vi "GrabFullListing.vi"(10 "Device In":T1, 11 "MulticolumnListbox in":refnum<vi>) -> (2 "tags":string[](array[string]))   [LabVIEW 2016, in "Systemlink Tag.xctl"]
uses:
  <userlib>/MicroPython/VIs/SystemLink/Systemlink Tag.xctl
  <userlib>/MicroPython/VIs/SystemLink/SkylineCluster.ctl
panel:
  out "Table Control":string[][](table)
  out "error out":errorcluster
  in  "error in":errorcluster
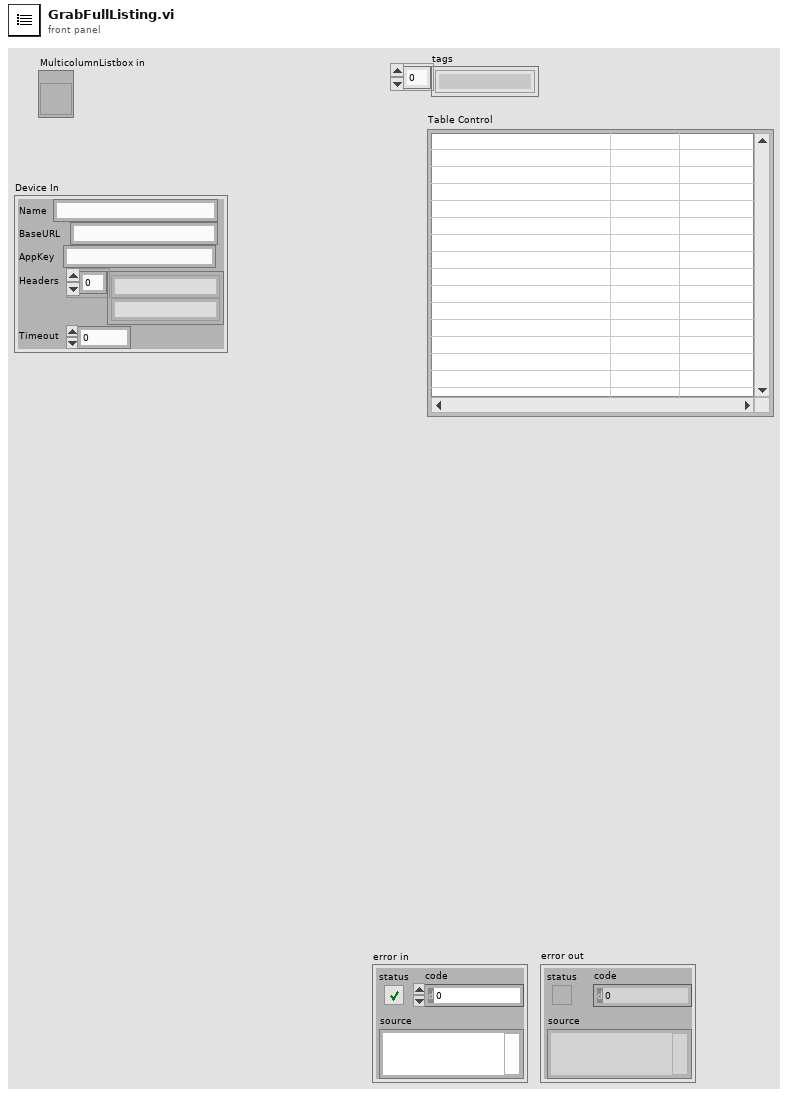
[diagram p1: front panel]
types:
  T1 = typedef "SkylineCluster.ctl" = cluster{"Name":string, "BaseURL":string, "AppKey":string, "Headers":string[], "Timeout":i32}
  T2 = cluster{"tagsWithValues":cluster{"tag":cluster{"path":string, "type":string}, "current":cluster{"timestamp":string, "value":cluster{"type":string, "value":string}}}[]}
  T3 = typedef "SystemLinkHTTPComm.ctl" = cluster{"url":string, "sent headers":string, "sent body":string, "headers":string, "body":string, "Sent":string, "Received":string}
  T4 = cluster{"tag":cluster{"path":string, "type":string}, "current":cluster{"timestamp":string, "value":cluster{"type":string, "value":string}}}[]
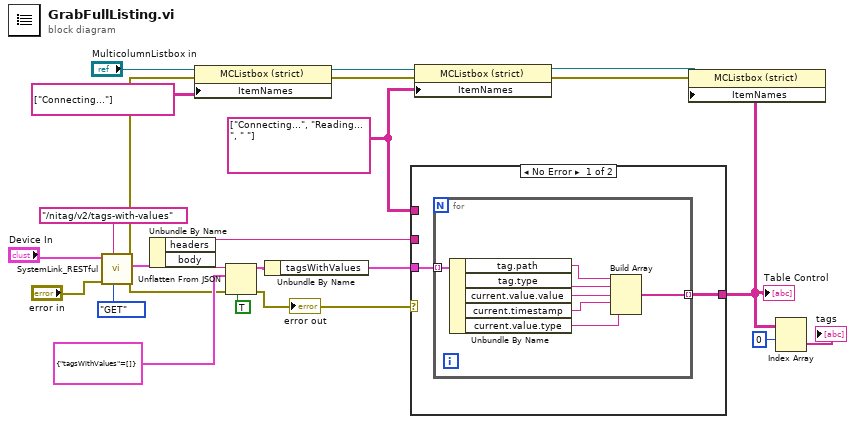
[diagram p0: block diagram]
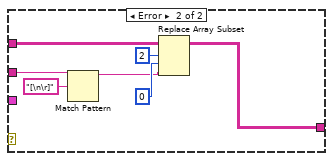
[diagram p2: hidden frame]
diagram:
  w1 = string[][] [["Connecting..."], ["Reading..."], [" "]] ("Item Names")
  n1 = call <userlib>:"SystemLink_RESTful.vi"("Method"=enum16{"GET", "PUT", "POST", "MultiPOST"}."GET", "url"="/nitag/v2/tags-with-values", "error in"="error in", "Device In"="Device In") -> ("error out"=w9:errorcluster, "Comm"=w20:T3)  [unwired: 4 in, 2 out]
  n2 = Unbundle By Name(w20) -> ("headers"=w2:string, "body"=w10:string)
  n3 = property on="Property Node" class="MCListbox (strict)"(reference="MulticolumnListbox in", "ItemNames"=string[][] [["Connecting..."]] ("Item Names")) -> (reference out=w11:refnum<vi>)  [unwired: 1 in, 1 out]
  n4 = Unflatten From JSON(JSON string=w10, type and defaults=T2 {"tagsWithValues"=[]}, default null elements? (F)=TRUE, error in (no error)=w9) -> (value=w19:T2, error out=w3:errorcluster)  [unwired: 3 in]
  "error out" <- w3
  n5 = Unbundle By Name(w19) -> ("tagsWithValues"=w14:T4)
  n6 = case shown="No Error" w3 {
    tunnel: w14 -> [w24 _]
    tunnel: [w23 w32] -> w7
    tunnel: w2 -> [_ w38]
    tunnel: w1 -> [_ w36]
    frame No Error {
      n7 = for {
        tunnel: w24 -> [w31] mode=indexing
        tunnel: [w26] -> w23 mode=indexing
        n8 = Unbundle By Name(w31) -> ("tag.path"=w25:string, "tag.type"=w30:string, "current.value.value"=w29:string, "current.timestamp"=w28:string, "current.value.type"=w27:string)
        n9 = Build Array(w25, w30, w29, w28, w27) -> (w26:string[])
      }
    }
    frame Error {
      n10 = Match Pattern(string=w38, regular expression="[\n\r]") -> (before substring=w33:string)  [unwired: 1 in, 3 out]
      n11 = Replace Array Subset(array=w36, new element=w33, index (row)=2, index (col)=0 ("disabled index (col)")) -> (w32:string[][])
    }
  }
  "Table Control" <- w7
  n12 = property on="Property Node" class="MCListbox (strict)"(reference=w11, error in=w9, "ItemNames"=w1) -> (reference out=w8:refnum<vi>, error out=w4:errorcluster)
  n13 = property on="Property Node" class="MCListbox (strict)"(reference=w8, error in=w4, "ItemNames"=w7) -> ()  [unwired: 2 out]
  n14 = Index Array(array=w7, index (row)=0) -> (element=→"tags":string[])  [unwired: 1 in]
